vi "Recorder.vi"() -> ()   [LabVIEW 2014]
uses:
  <vilib>/express/express arith-compare/Formula/XNode/ExpressFormulaBlockNode.xnode
panel:
  in  "device name":tag="myDAQ1"
  out "?":u8(slide) scale=0.0..100.0
  in  "stop":bool
  in  "Start Recording":bool
  out "data":dynamicdata(graph) caption="Sound Waveform"
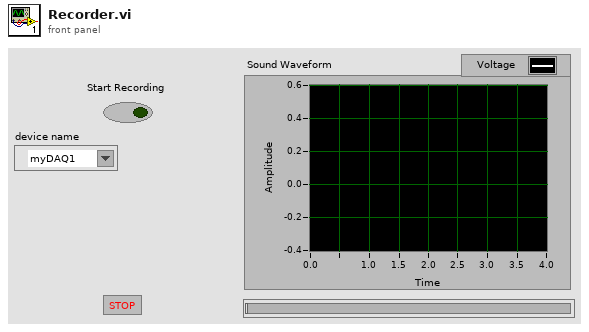
[diagram p1: front panel]
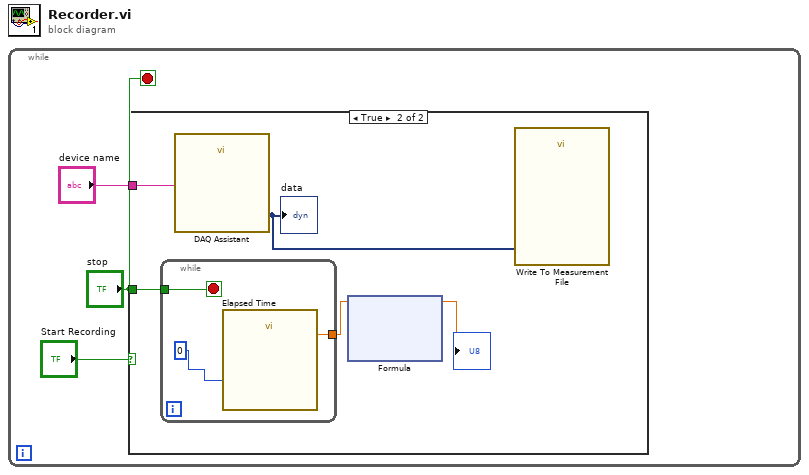
[diagram p0: block diagram]
diagram:
  n1 = while {
    stop <- "stop" stop-if-true
    n2 = case shown="True" "Start Recording" {
      tunnel: "stop" -> [_ w8]
      tunnel: "device name" -> [_ w4]
      frame False {
      }
      frame True {
        n3 = while {
          tunnel: w8 -> [w19]
          tunnel: [w18] -> w7
          stop <- w19 stop-if-true
          n4 = call "Elapsed Time"("Set Start Time (s)"=0) -> ("Elapsed Time (s)"=w18:dbl)  [unwired: 11 in, 7 out]
        }
        n5 = call "DAQ Assistant"("device name"=w4) -> ("data"=w5:dynamicdata)  [unwired: 16 in, 2 out]
        "data" <- w5
        n6 = xnode "Formula"("X1"=w7) -> ("Result"=→"?":dbl)  [unwired: 1 in, 1 out]
        n7 = call "Write To Measurement File"("Signals"=w5) -> ()  [unwired: 16 in, 3 out]
      }
    }
  }
